vi "Rearrange elements in 2 darray.vi"(9 "Pretransform Rubix Array":T1[][](array[typedef]), 10 "To":cluster{"row":i32, "column":i32}[](array[cluster]), 11 "From":cluster{"row":i32, "column":i32}[](array[cluster])) -> (1 "Transform Rubix Array":T1[][](array[typedef]), 2 "Facets to move":T1[](array[typedef]))   [LabVIEW 2019]
uses:
  Rubix Array data type.ctl
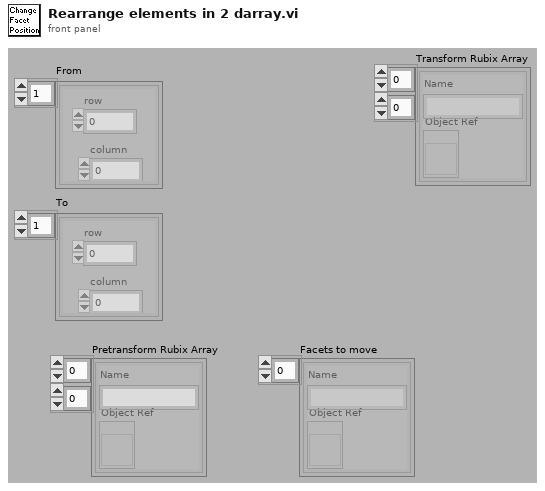
[diagram p1: front panel]
types:
  T1 = typedef "Rubix Array data type.ctl" = cluster{"Object Ref":refnum<vi>, "Name":string}
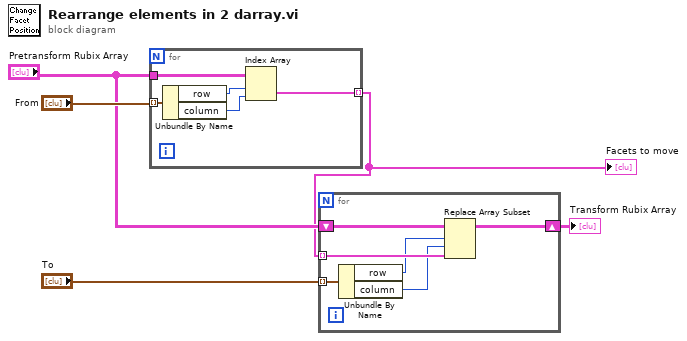
[diagram p0: block diagram]
diagram:
  n1 = for {
    tunnel: "From" -> [w9] mode=indexing
    tunnel: "Pretransform Rubix Array" -> [w10]
    tunnel: [w6] -> w2 mode=indexing
    n2 = Unbundle By Name(w9) -> ("row"=w8:i32, "column"=w7:i32)
    n3 = Index Array(array=w10, index (row)=w8, index (col)=w7) -> (element=w6:T1)
  }
  "Facets to move" <- w2
  n4 = for {
    shift-right: [w11] -> w1
    shift-left: "Pretransform Rubix Array" -> [w16]
    tunnel: "To" -> [w15] mode=indexing
    tunnel: w2 -> [w14] mode=indexing
    n5 = Unbundle By Name(w15) -> ("row"=w13:i32, "column"=w12:i32)
    n6 = Replace Array Subset(array=w16, new element=w14, index (row)=w13, index (col)=w12) -> (w11:T1[][])
  }
  "Transform Rubix Array" <- w1
